vi "UTILITY Write Header.vi"(7 "Array Type":enum16{"1D", "2D"}(ring), 8 "error in (no error)":errorcluster, 9 "Headers 2D":string[][](array[string])=[["Date", "Time", "APP Version", "XML Version", "Daily Build", "Machine State", "Motor Profile", "Motor Profile Status", "Motor Mode", "Cycle Selected", "Cycle Engine Status", "Temperature (F)", "Lid Status", "Basket Speed (RPM)", "Motor Current RMS (AMPS)", "Tub Volume (Gal)", "Pressure (in H2O)", "Lid Lock Status", "Mode Shift Status", "Hot Water Valve", "Cold Water Valve", "Spray/Rinse Valve", "Fabric Softener Valve", "Drain Pump", "Recirculation Pump", "Sub-Cycle", "Cycle Count", "Shaft Speed", "ME Relay", "Valve Relay", "MS Motor", "Deep Fill", "Warm Rinse", "Deep Rinse/FS", "My Cycle", "Extra Rinse", "Temp Level", "Soil Level", "Spin Level", "Load Size", "Stain", "Delay Time", "Soak Time", "Auto Soak Level", "Dry Load Size", "Wet Load Gallons", "Target Gallons", "Load Type", "Target Level (inches)", "Mode Shift Feedback", "Red. Version", "Red. Pressure", "Red. Shaft Speed", "Red. Mode Shift FB", "Red. Lid Switch", "Red. Lid Lock", "Red. Motor Enable", "Red. Triac Enable", "Red. Drain Pump", "Red. Lid Lock  Speed Interlock", "Red. Flood State", "Red. Lid Open  Fault State", "Red. Unlock Fault State", "Red. Access to Moving Parts", "Redundant Heartbeat", "Segment Gallons", "Target Bath Temp (F)", "Current Bath Temp (F)", "ERD 1", "ERD 2", "ERD 3", "Lid Lock FB", "Hot Gallons", "Cold Gallons", "Hot Inlet Temp", "Cold Inlet temp", "Warm Inlet Temp", "Hot Seg Valve Time", "Cold Seg Valve Time", "Coast Time", "Ramp Time", "Ramp Speed", "Ramp Avg Current", "Partial Coast Time", "Dry Load Size", "Ramp Line Voltage", "Coast Line Voltage", "Lid Lock Req State", "OOB Det in Accel", "Max Accel in Accel", "Max Jerk in Accel", "OOB det in S-S", "Max Jerk in S-S", "OOB Redist Req", "Remaining Cycle Time (s)"]], 10 "Headers":string[](array[string])=["Date", "Time", "APP Version", "XML Version", "Daily Build", "Machine State", "Motor Profile", "Motor Profile Status", "Motor Mode", "Cycle Selected", "Cycle Engine Status", "Temperature (F)", "Lid Status", "Basket Speed (RPM)", "Motor Current RMS (AMPS)", "Tub Volume (Gal)", "Pressure (in H2O)", "Lid Lock Status", "Mode Shift Status", "Hot Water Valve", "Cold Water Valve", "Spray/Rinse Valve", "Fabric Softener Valve", "Drain Pump", "Recirculation Pump", "Sub-Cycle", "Cycle Count", "Shaft Speed", "ME Relay", "Valve Relay", "MS Motor", "Deep Fill", "Warm Rinse", "Deep Rinse/FS", "My Cycle", "Extra Rinse", "Temp Level", "Soil Level", "Spin Level", "Load Size", "Stain", "Delay Time", "Soak Time", "Auto Soak Level", "Dry Load Size", "Wet Load Gallons", "Target Gallons", "Load Type", "Target Level (inches)", "Mode Shift Feedback", "Red. Version", "Red. Pressure", "Red. Shaft Speed", "Red. Mode Shift FB", "Red. Lid Switch", "Red. Lid Lock", "Red. Motor Enable", "Red. Triac Enable", "Red. Drain Pump", "Red. Lid Lock  Speed Interlock", "Red. Flood State", "Red. Lid Open  Fault State", "Red. Unlock Fault State", "Red. Access to Moving Parts", "Redundant Heartbeat", "Segment Gallons", "Target Bath Temp (F)", "Current Bath Temp (F)", "ERD 1", "ERD 2", "ERD 3", "Lid Lock FB", "Hot Gallons", "Cold Gallons", "Hot Inlet Temp", "Cold Inlet temp", "Warm Inlet Temp", "Hot Seg Valve Time", "Cold Seg Valve Time", "Coast Time", "Ramp Time", "Ramp Speed", "Ramp Avg Current", "Partial Coast Time", "Dry Load Size", "Ramp Line Voltage", "Coast Line Voltage", "Lid Lock Req State", "OOB Det in Accel", "Max Accel in Accel", "Max Jerk in Accel", "OOB det in S-S", "Max Jerk in S-S", "OOB Redist Req", "Remaining Cycle Time (s)"], 11 "File Path Control":path) -> (0 "error out":errorcluster, 3 "Byte Stream File out":refnum<file>)   [LabVIEW 2016]
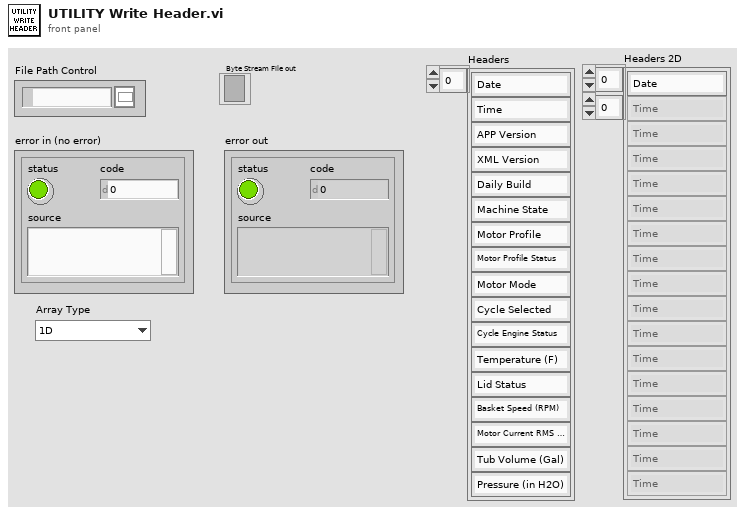
[diagram p1: front panel]
types:
  T1 = enum16{"open", "replace", "create", "open or create", "replace or create", "replace or create with confirmation"}
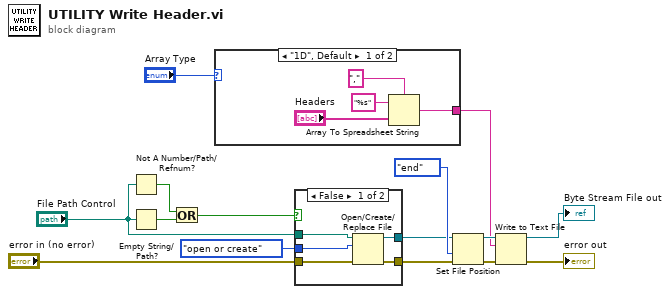
[diagram p0: block diagram]
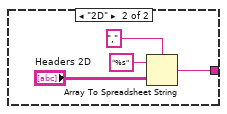
[diagram p2: hidden frame]
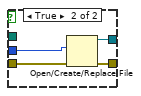
[diagram p3: hidden frame]
diagram:
  n1 = Not A Number/Path/Refnum?(number/path/refnum="File Path Control") -> (NaN/Path/Refnum?=w11:bool)
  n2 = Empty String/Path?(string/path="File Path Control") -> (empty?=w10:bool)
  n3 = Or(x=w11, y=w10) -> (x .or. y?=w9:bool)
  n4 = case shown="\"1D\", Default" "Array Type" {
    tunnel: [w16 w20] -> w1
    frame "1D", Default {
      n5 = Array To Spreadsheet String(delimiter (Tab)=",", array="Headers", 3:"%s" ("format string")) -> (spreadsheet string=w16:string)
    }
    frame "2D" {
      n6 = Array To Spreadsheet String(delimiter (Tab)=",", array="Headers 2D", 3:"%s" ("format string")) -> (spreadsheet string=w20:string)
    }
  }
  n7 = case shown="False" w9 {
    tunnel: T1."open or create" ("operation (0:open)") -> [w26 w32]
    tunnel: [w27 w31] -> w4
    tunnel: "File Path Control" -> [w28 _]
    tunnel: "error in (no error)" -> [w25 w30]
    tunnel: [w24 w29] -> w7
    frame False {
      n8 = Open/Create/Replace File(file path (use dialog)=w28, error in=w25, operation (0:open)=w26) -> (refnum out=w27:refnum<file>, error out=w24:errorcluster)  [unwired: 3 in, 1 out]
    }
    frame True {
      n9 = Open/Create/Replace File(error in=w30, operation (0:open)=w32) -> (refnum out=w31:refnum<file>, error out=w29:errorcluster)  [unwired: 4 in, 1 out]
    }
  }
  n10 = Set File Position(refnum=w4, from (0:start)=enum16{"start", "end", "current"}."end", error in=w7) -> (refnum out=w3:refnum<file>, error out=w6:errorcluster)  [unwired: 1 in]
  n11 = Write to Text File(file (use dialog)=w3, text=w1, error in=w6) -> (refnum out=→"Byte Stream File out":refnum<file>, error out=→"error out":errorcluster)  [unwired: 1 in, 1 out]
